vi "Construct Field by Parsing Ctrl Label.vi"(8 "error in (no error)":errorcluster, 11 "FK Ring in":refnum<class "FK Ring.lvclass">) -> (0 "error out":errorcluster, 3 "FK Ring out":refnum<class "FK Ring.lvclass">)   [LabVIEW 2020, in "FK Ring.lvclass"]
uses:
  FK Ring.lvclass
  Ring Field.lvclass
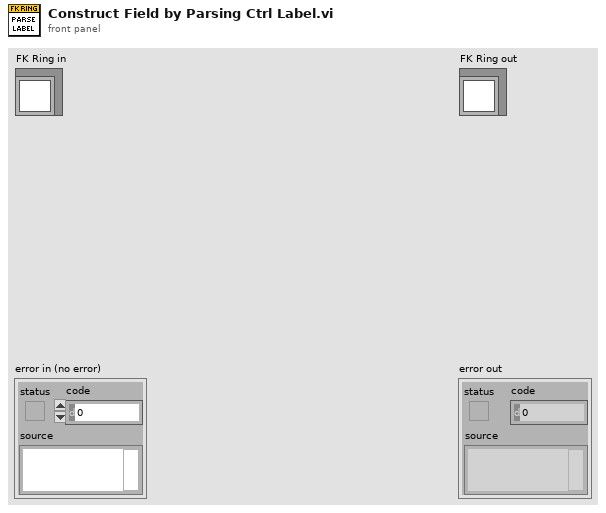
[diagram p1: front panel]
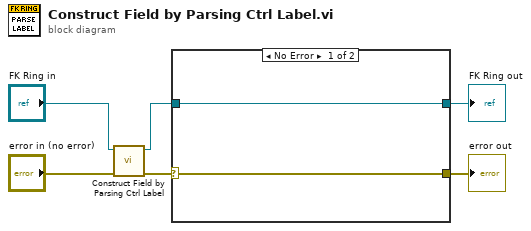
[diagram p0: block diagram]
diagram:
  n1 = call-parent "Construct Field by Parsing Ctrl Label.vi"("error in (no error)"="error in (no error)", "Field in"="FK Ring in") -> ("error out"=w4:errorcluster, "Field out"=w3:refnum<class "FK Ring.lvclass">)  [unwired: 8 in]
  n2 = case shown="No Error" w4 {
    selector: w4 -> [w8 w9]
    tunnel: w3 -> [w7 w10]
    tunnel: [w7 w10] -> w2
    tunnel: [w8 w9] -> w1
    frame No Error {
    }
    frame Error {
    }
  }
  "error out" <- w1
  "FK Ring out" <- w2
